vi "Filter Duplicate Images out.vi"(8 "Error In":errorcluster, 9 "GreyLevel Drops and time Derivative in":dbl[][](array[numeric]), 10 "GreyLevel Drops and time in":dbl[][](array[numeric]), 11 "Rel Time (s) in":u32[](array[numeric])) -> (0 "Error Out":errorcluster, 1 "GreyLevel Drops and time Derivative out":dbl[][](array[numeric]), 2 "GreyLevel Drops and time out":dbl[][](array[numeric]), 3 "Rel Time (s) out":u32[](array[numeric]))   [LabVIEW 2013]
panel:
  # "Filters Duplicate images by checking when the derivative is zero"
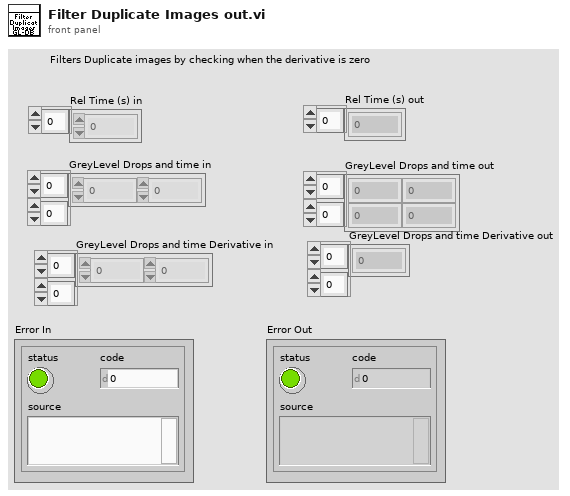
[diagram p1: front panel]
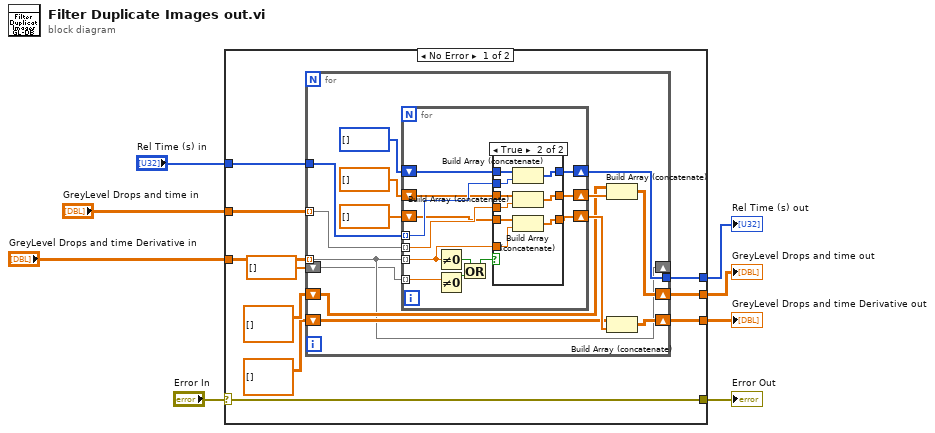
[diagram p0: block diagram]
diagram:
  n1 = case shown="No Error" "Error In" {
    selector: "Error In" -> [w18 w61]
    tunnel: [w18 w61] -> w7
    tunnel: [w10 w60] -> w6
    tunnel: "Rel Time (s) in" -> [w17 w60]
    tunnel: [w14 w59] -> w4
    tunnel: "GreyLevel Drops and time in" -> [w16 w59]
    tunnel: [w13 w58] -> w2
    tunnel: "GreyLevel Drops and time Derivative in" -> [w15 w58]
    frame No Error {
      n2 = for {
        tunnel: w17 -> [w31]
        tunnel: w16 -> [w32] mode=indexing
        tunnel: w15 -> [w20] mode=indexing
        shift-right: [w27] -> w14
        shift-left: dbl[][] [] -> [w26]
        shift-right: [w28] -> w13
        shift-left: dbl[][] [] -> [w25]
        tunnel: [w21] -> w10
        shift-right: [w20] -> _
        shift-left: dbl[] [] ("GreyLevel Drops and time Derivative in") -> [w19]
        n3 = for {
          tunnel: w20 -> [w45] mode=indexing
          tunnel: w32 -> [w44] mode=indexing
          tunnel: w31 -> [w43] mode=indexing
          shift-right: [w42] -> w21
          shift-left: u32[] [] -> [w41]
          shift-right: [w39] -> w29
          shift-left: dbl[] [] -> [w37]
          shift-right: [w40] -> w30
          shift-left: dbl[] [] -> [w38]
          tunnel: w19 -> [w36] mode=indexing
          n4 = Not Equal To 0?(x=w45) -> (x != 0?=w35:bool)
          n5 = Not Equal To 0?(x=w36) -> (x != 0?=w34:bool)
          n6 = Or(x=w35, y=w34) -> (x .or. y?=w33:bool)
          n7 = case shown="True" w33 {
            tunnel: w45 -> [_ w57]
            tunnel: w44 -> [_ w56]
            tunnel: w43 -> [_ w55]
            tunnel: [w48 w54] -> w42
            tunnel: w41 -> [w48 w53]
            tunnel: [w47 w52] -> w40
            tunnel: [w46 w51] -> w39
            tunnel: w38 -> [w47 w50]
            tunnel: w37 -> [w46 w49]
            frame False {
            }
            frame True {
              n8 = Build Array (concatenate)(w53, w55) -> (w54:u32[])
              n9 = Build Array (concatenate)(w50, w56) -> (w52:dbl[])
              n10 = Build Array (concatenate)(w49, w57) -> (w51:dbl[])
            }
          }
        }
        n11 = Build Array (concatenate)(w26, w30) -> (w27:dbl[][])
        n12 = Build Array (concatenate)(w25, w29) -> (w28:dbl[][])
      }
    }
    frame Error {
    }
  }
  "Error Out" <- w7
  "Rel Time (s) out" <- w6
  "GreyLevel Drops and time out" <- w4
  "GreyLevel Drops and time Derivative out" <- w2
